vi "ErrorDisplay.vi"(5 "eDialogType":T1(ring), 7 "Warning (f)":bool, 8 "Details":string, 9 "Source":string, 10 "Length":i32[](array[numeric]), 11 "Start":i32[](array[numeric])) -> (1 "bStop":bool, 2 "bAbort":bool, 3 "bContinue":bool)   [LabVIEW 2014, in "NISTErrorLib.lvlib"]
uses:
  NISTErrorLib.lvlib
  <vilib>/Utility/error.llb/ErrWarn.ctl
  <vilib>/Utility/miscctls.llb/LVKeyNavTypeDef.ctl
panel:
  in  "btnAbort":bool
  in  "btnContinue":bool
  in  "btnStop":bool
  out "DetailPane":string
  out "ErrorOrWarningGlyph":T2
  out "Source of Error":string
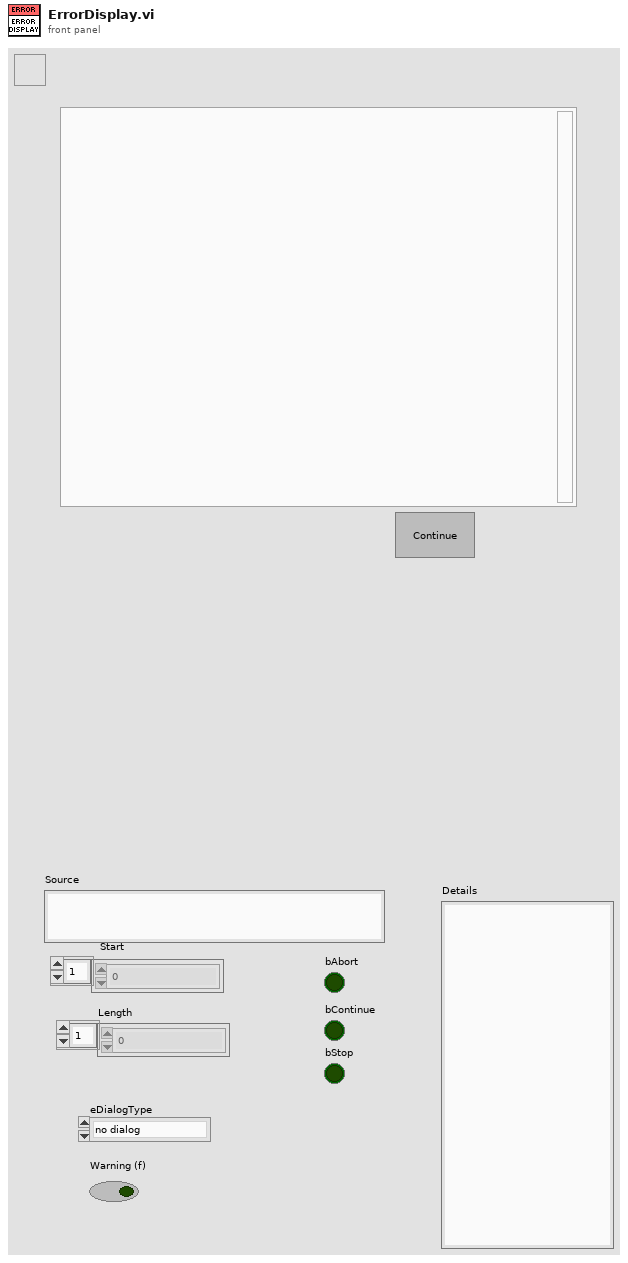
[diagram p1: front panel]
types:
  T1 = enum16{"no dialog", "Continue", "Continue Stop", "Abort Continue Stop", "Stop"}
  T2 = typedef "ErrWarn.ctl" = bool
  T3 = typedef "LVKeyNavTypeDef.ctl" = cluster{"Control":bool, "Shift":bool, "Key":string}
  T4 = enum32{"Invalid", "Standard", "Closed", "Hidden", "Minimized", "Maximized"}
  T5 = typedef "LVRectTypeDef.ctl" = cluster{"Left":i16, "Top":i16, "Right":i16, "Bottom":i16}
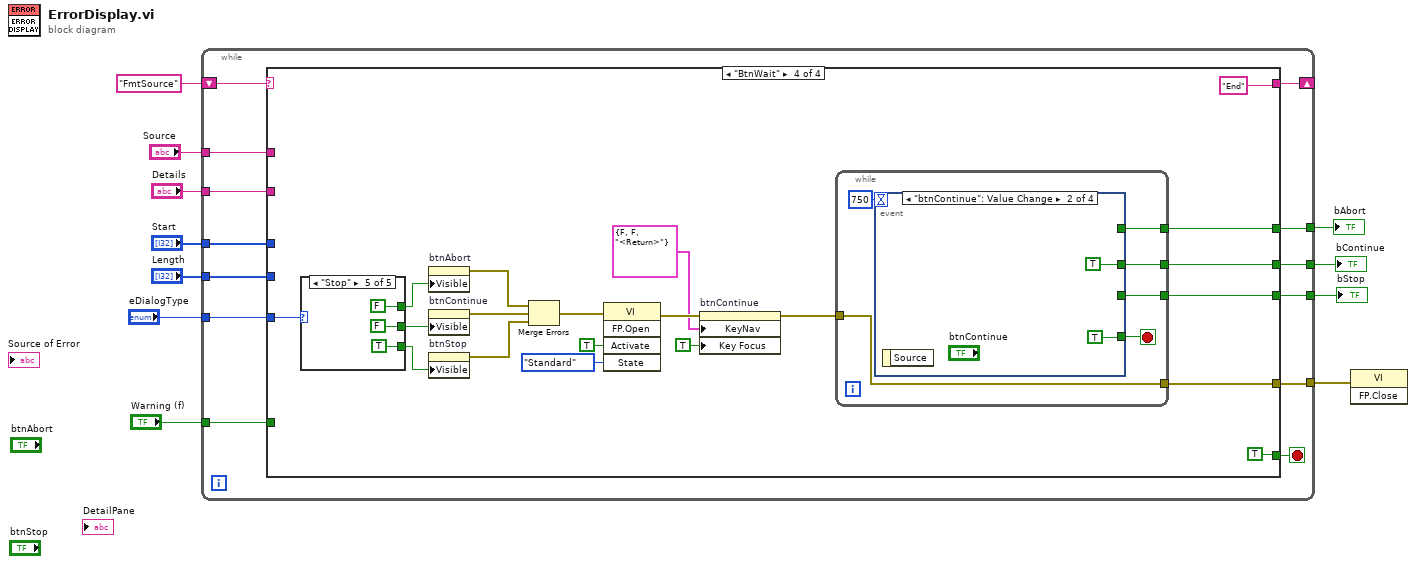
[diagram p0: block diagram]
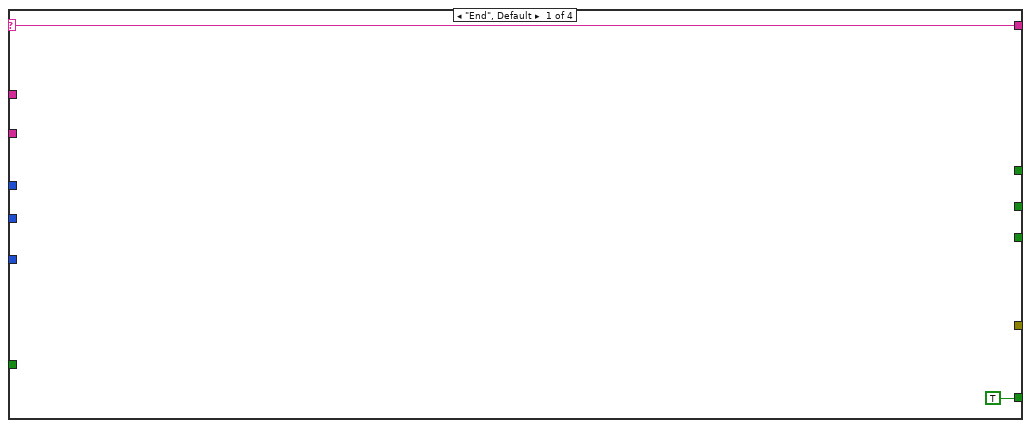
[diagram p2: hidden frame]
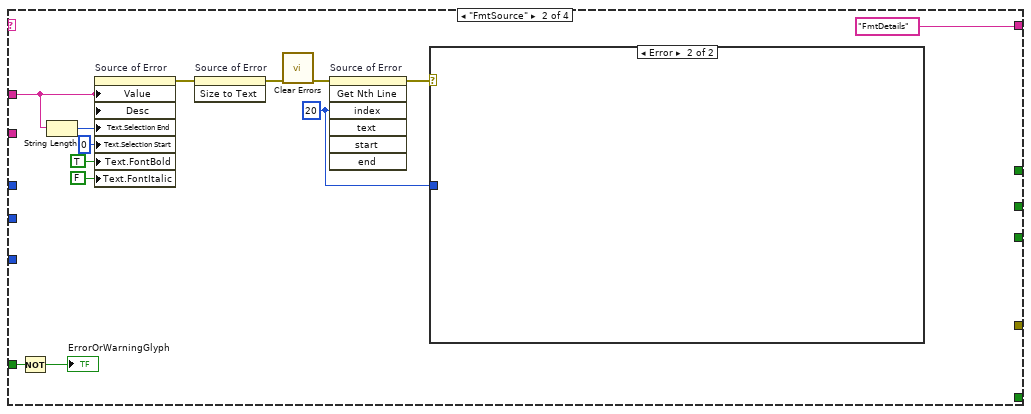
[diagram p3: hidden frame]
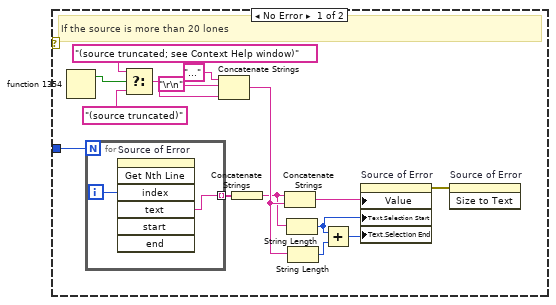
[diagram p4: hidden frame]
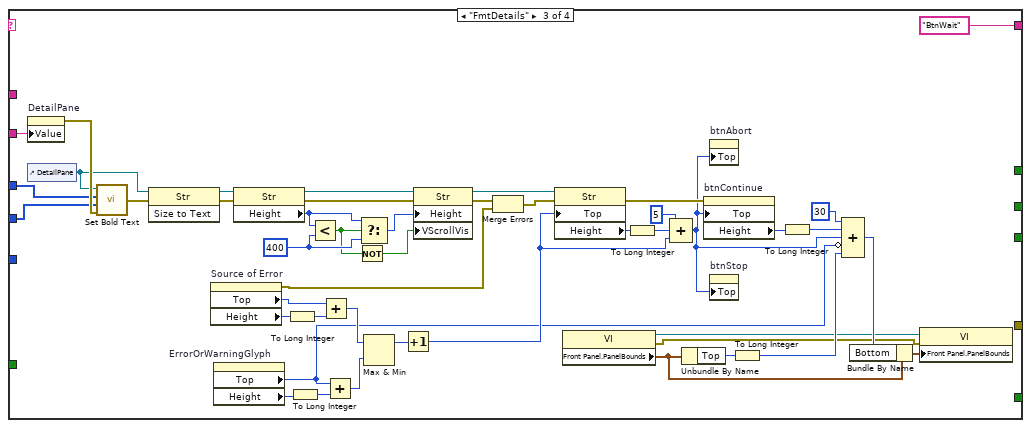
[diagram p5: hidden frame]
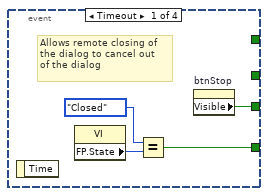
[diagram p6: hidden frame]
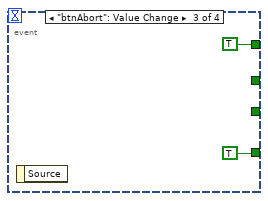
[diagram p7: hidden frame]
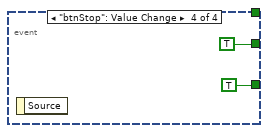
[diagram p8: hidden frame]
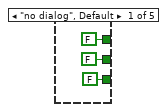
[diagram p9: hidden frame]
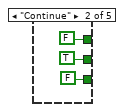
[diagram p10: hidden frame]
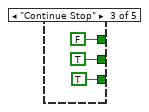
[diagram p11: hidden frame]
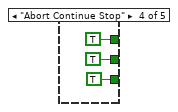
[diagram p12: hidden frame]
diagram:
  n1 = while {
    shift-right: [w21] -> _
    shift-left: "FmtSource" -> [w24]
    tunnel: "Source" -> [w23]
    tunnel: "Details" -> [w20]
    tunnel: "Start" -> [w19]
    tunnel: "Length" -> [w18]
    tunnel: "eDialogType" -> [w17]
    tunnel: [w16] -> w5
    tunnel: [w15] -> w4
    tunnel: [w14] -> w3
    tunnel: "Warning (f)" -> [w13]
    tunnel: [w12] -> w1
    stop <- w22 stop-if-true
    n2 = case shown="\"BtnWait\"" w24 {
      selector: w24 -> [w25 _ _ _]
      tunnel: w23 -> [_ w37 _ _]
      tunnel: [TRUE _ _ TRUE] -> w22
      tunnel: [w25 "FmtDetails" "BtnWait" "End"] -> w21
      tunnel: w20 -> [_ _ w101 _]
      tunnel: w19 -> [_ _ w93 _]
      tunnel: w18 -> [_ _ w92 _]
      tunnel: w17 -> [_ _ _ w121]
      tunnel: [_ _ _ w107] -> w16
      tunnel: [_ _ _ w106] -> w15
      tunnel: [_ _ _ w105] -> w14
      tunnel: w13 -> [_ w28 _ _]
      tunnel: [_ _ _ w102] -> w12
      frame "End", Default {
      }
      frame "FmtSource" {
        w29 = u32 20 ("line index")
        n3 = Not(x=w28) -> (.not. x?=→"ErrorOrWarningGlyph":bool)
        n4 = String Length(string=w37) -> (length=w38:i32)
        n5 = property on="Source of Error" class="Str"("Value"=w37, "Desc"=w37, "Text.Selection End"=w38, "Text.Selection Start"=u32 0 ("Text.Selection:Start"), "Text.FontBold"=TRUE ("Text.Font:Bold"), "Text.FontItalic"=FALSE ("Text.Font:Italic")) -> (error out=w33:errorcluster)  [unwired: 2 in, 1 out]
        n6 = invoke on="Source of Error" class="Str" method="Size to Text"(error in=w33) -> (error out=w32:errorcluster)  [unwired: 2 in, 2 out]
        n7 = call <vilib>:"Clear Errors.vi"("error in (no error)"=w32) -> ("error out"=w31:errorcluster)  [unwired: 5 in, 1 out]
        n8 = invoke on="Source of Error" class="Str" method="Get Nth Line"(error in=w31, "index"=w29) -> (error out=w30:errorcluster)  [unwired: 5 in, 6 out]
        n9 = case shown="Error" w30 {
          tunnel: w29 -> [w40 _]
          frame No Error {
            # "If the source is more than 20 lones"
            n10 = fn#1354() -> (1:w54:bool)  [unwired: 1 out]
            n11 = for {
              N: w40 -> [_]
              tunnel: [w55] -> w46 mode=indexing
              i -> [w56]
              n12 = invoke on="Source of Error" class="Str" method="Get Nth Line"("index"=w56) -> ("text"=w55:string)  [unwired: 6 in, 6 out]
            }
            n13 = Select(t="(source truncated; see Context Help window)", s=w54, f="(source truncated)") -> (s? t:f=w51:string)
            n14 = Concatenate Strings("...", "\r\n", w51) -> (w48:string)
            n15 = Concatenate Strings(w46) -> (w45:string)
            n16 = Concatenate Strings(w45, w48) -> (w44:string)
            n17 = String Length(string=w45) -> (length=w43:i32)
            n18 = String Length(string=w48) -> (length=w47:i32)
            n19 = Add(x=w43, y=w47) -> (x+y=w42:i32)
            n20 = property on="Source of Error" class="Str"("Value"=w44, "Text.Selection Start"=w43, "Text.Selection End"=w42) -> (error out=w41:errorcluster)  [unwired: 2 in, 1 out]
            n21 = invoke on="Source of Error" class="Str" method="Size to Text"(error in=w41) -> ()  [unwired: 2 in, 3 out]
          }
          frame Error {
          }
        }
      }
      frame "FmtDetails" {
        w89 = 400
        n22 = property on="DetailPane" class="Str"("Value"=w101) -> (error out=w100:errorcluster)  [unwired: 2 in, 1 out]
        n23 = control-ref of="DetailPane"() -> (w99:refnum<vi>)
        n24 = call <vilib>:"Set Bold Text.vi"("error in"=w100, "Length"=w92, "Start"=w93, "text"=w99) -> ("error out"=w98:errorcluster)  [unwired: 2 in]
        n25 = invoke class="Str" method="Size to Text"(reference=w99, error in=w98) -> (reference out=w96:refnum<vi>, error out=w95:errorcluster)  [unwired: 1 in, 1 out]
        n26 = property on="Source of Error" class="Str"() -> (error out=w76:errorcluster, "Top"=w82:i32, "Height"=w85:u32)  [unwired: 2 in, 1 out]
        n27 = property on="ErrorOrWarningGlyph" class="Bool"() -> ("Top"=w64:i32, "Height"=w84:u32)  [unwired: 2 in, 2 out]
        n28 = property class="Str"(reference=w96, error in=w95) -> (reference out=w94:refnum<vi>, error out=w91:errorcluster, "Height"=w90:u32)
        n29 = To Long Integer(number=w85) -> (32bit integer=w83:i32)
        n30 = To Long Integer(number=w84) -> (32bit integer=w81:i32)
        n31 = Less?(x=w90, y=w89) -> (x < y?=w88:bool)
        n32 = Add(x=w82, y=w83) -> (x+y=w79:i32)
        n33 = Add(x=w64, y=w81) -> (x+y=w80:i32)
        n34 = Not(x=w88) -> (.not. x?=w86:bool)
        n35 = Select(t=w90, s=w88, f=w89) -> (s? t:f=w87:u32)
        n36 = Max & Min(x=w79, y=w80) -> (max(x,y)=w78:i32)  [unwired: 1 out]
        n37 = Increment(x=w78) -> (x+1=w71:i32)
        n38 = property class="Str"(reference=w94, error in=w91, "Height"=w87, "VScrollVis"=w86) -> (reference out=w74:refnum<vi>, error out=w77:errorcluster)
        n39 = Merge Errors(w77, w76) -> (w75:errorcluster)
        n40 = property class="Str"(reference=w74, error in=w75, "Top"=w71) -> (error out=w70:errorcluster, "Height"=w73:u32)  [unwired: 1 out]
        n41 = property class="VI"() -> (reference out=w57:refnum<vi>, error out=w60:errorcluster, "Front Panel.PanelBounds"=w59:T5)  [unwired: 2 in]
        n42 = To Long Integer(number=w73) -> (32bit integer=w72:i32)
        n43 = Compound Arithmetic op=ADD(5 ("value"), w72, w71) -> (w67:i32)
        n44 = Unbundle By Name(w59) -> ("Top"=w65:i16)
        n45 = property on="btnContinue" class="Bool"(error in=w70, "Top"=w67) -> ("Height"=w69:u32)  [unwired: 1 in, 2 out]
        n46 = property on="btnAbort" class="Bool"("Top"=w67) -> ()  [unwired: 2 in, 2 out]
        n47 = property on="btnStop" class="Bool"("Top"=w67) -> ()  [unwired: 2 in, 2 out]
        n48 = To Long Integer(number=w65) -> (32bit integer=w63:i32)
        n49 = To Long Integer(number=w69) -> (32bit integer=w68:i32)
        n50 = Compound Arithmetic op=ADD(30 ("value"), w68, w67, invert w64, w63) -> (w62:i32)
        n51 = Bundle By Name(cluster=w59, "Bottom"=w62) -> (w58:T5)
        n52 = property class="VI"(reference=w57, error in=w60, "Front Panel.PanelBounds"=w58) -> ()  [unwired: 2 out]
      }
      frame "BtnWait" {
        n53 = case shown="\"Stop\"" w121 {
          tunnel: [FALSE FALSE FALSE TRUE FALSE] -> w118
          tunnel: [FALSE TRUE TRUE TRUE FALSE] -> w120
          tunnel: [FALSE FALSE TRUE TRUE TRUE] -> w119
          frame "no dialog", Default {
          }
          frame "Continue" {
          }
          frame "Continue Stop" {
          }
          frame "Abort Continue Stop" {
          }
          frame "Stop" {
          }
        }
        n54 = property on="btnAbort" class="Bool"("Visible"=w118) -> (error out=w117:errorcluster)  [unwired: 2 in, 1 out]
        n55 = property on="btnContinue" class="Bool"("Visible"=w120) -> (error out=w116:errorcluster)  [unwired: 2 in, 1 out]
        n56 = property on="btnStop" class="Bool"("Visible"=w119) -> (error out=w115:errorcluster)  [unwired: 2 in, 1 out]
        n57 = Merge Errors(w117, w116, w115) -> (w112:errorcluster)
        n58 = invoke class="VI" method="FP.Open"(error in=w112, "Activate"=TRUE ("Activate?"), "State"=T4."Standard") -> (error out=w111:errorcluster)  [unwired: 2 in, 4 out]
        n59 = property on="btnContinue" class="Bool"(error in=w111, "KeyNav"=T3 {"Control"=FALSE, "Shift"=FALSE, "Key"="<Return>"} ("Focus Key Binding"), "Key Focus"=TRUE) -> (error out=w108:errorcluster)  [unwired: 1 in, 1 out]
        n60 = while {
          tunnel: w108 -> [w122]
          tunnel: [w126] -> w107
          tunnel: [w124] -> w106
          tunnel: [w123] -> w105
          tunnel: [w122] -> w102
          stop <- w125 stop-if-true
          n61 = event shown="[1] \"btnContinue\": Value Change" {
            selector: _ -> [_ _ _ _]
            dyn-events: _ -> [_ _ _ _]
            timeout: 750 -> [_ _ _ _]
            tunnel: [w131 _ _ TRUE] -> w126
            tunnel: [w128 TRUE TRUE TRUE] -> w125
            tunnel: [_ TRUE _ _] -> w124
            tunnel: [_ _ TRUE _] -> w123
            event Timeout {
              # "Allows remote closing of\nthe dialog to cancel out \nof the dialog"
              n62 = event-data() -> ()  [unwired: 1 in, 1 out]
              n63 = property class="VI"() -> ("FP.State"=w130:T4)  [unwired: 2 in, 2 out]
              n64 = Equal?(x=T4."Closed" ("Front Panel Window:State"), y=w130) -> (x = y?=w128:bool)
              n65 = property on="btnStop" class="Bool"() -> ("Visible"=w131:bool)  [unwired: 2 in, 2 out]
            }
            event "btnContinue": Value Change {
              n66 = event-data() -> ()  [unwired: 1 in, 1 out]
            }
            event "btnAbort": Value Change {
              n67 = event-data() -> ()  [unwired: 1 in, 1 out]
            }
            event "btnStop": Value Change {
              n68 = event-data() -> ()  [unwired: 1 in, 1 out]
            }
          }
        }
      }
    }
  }
  "bStop" <- w5
  "bContinue" <- w4
  "bAbort" <- w3
  n69 = invoke class="VI" method="FP.Close"(error in=w1) -> ()  [unwired: 2 in, 3 out]
